vi "3Act Helper - RudderSettingToDynamixelDegrees.vi"(10 "Suggested Rudder Setpoint":T1 min=-1.0 max=1.0 scale=1.0..-1.0, 11 "Dynamixel Set Data":T2) -> (3 "Dynamixel Angle":dbl)   [LabVIEW 2013]
doc: "This VI takes in a -1 to 1 rudder setting and turns it into degree values for the Dynamixel. This is based strongly on the upper and lower bounds for the Dynamixel, which should be set from the OCU.\n\nEric Schneider, March 2014"
uses:
  Data/TypeDefs/DynamixelSetupInfo.ctl
  Data/TypeDefs/Rudder Set Suggestions.ctl
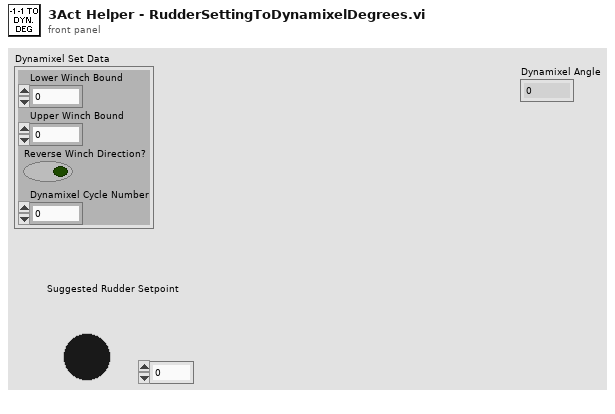
[diagram p1: front panel]
types:
  T1 = typedef "Rudder Set Suggestions.ctl" = dbl
  T2 = typedef "DynamixelSetupInfo.ctl" = cluster{"Lower Winch Bound":dbl, "Upper Winch Bound":dbl, "Reverse Winch Direction?":bool, "Dynamixel Cycle Number":i32}
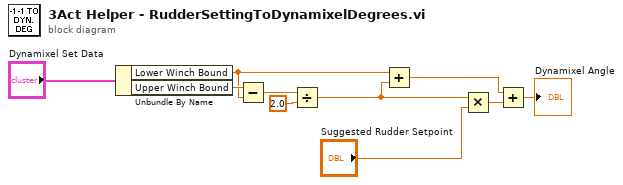
[diagram p0: block diagram]
diagram:
  n1 = Unbundle By Name("Dynamixel Set Data") -> ("Lower Winch Bound"=w1:dbl, "Upper Winch Bound"=w9:dbl)
  n2 = Subtract(x=w9, y=w1) -> (x-y=w5:dbl)
  n3 = Divide(x=w5, y=2.0) -> (x/y=w2:dbl)
  n4 = Add(x=w1, y=w2) -> (x+y=w3:dbl)
  n5 = Multiply(x=w2, y="Suggested Rudder Setpoint") -> (x*y=w8:T1)
  n6 = Add(x=w3, y=w8) -> (x+y=→"Dynamixel Angle":T1)
